vi "参数设置页.vi"() -> ()   [LabVIEW 2016, in "斯坦道总磷总氮.lvlib"]
uses:
  <vilib>/Plasmionique/MB Master/MB_Master/MB_Master.lvclass
  <vilib>/ptbypt/NI_PtbyPt.lvlib
panel:
  in  "简易流程周期设置":cluster{"switch button":bool, "设置按钮":bool}
  in  "维护模式":bool=TRUE
  out "连接状态":bool
  in  "标样核查自动补测":bool caption="通讯连接"
  in  "跨度核查自动补测":bool caption="通讯连接"
  in  "零点核查自动补测":bool caption="通讯连接"
  in  "标样核查标液偏差":dbl caption="标样核查标液偏差："
  in  "跨度核查标液偏差":dbl caption="跨度核查标液偏差："
  in  "零点核查标液偏差":dbl caption="零点核查标液偏差："
  out "低量程上限":dbl caption="低量程上限："
  in  "简易流程路径":path=path "data/流程.xml"
  out "数据刷新时间":string
  in  "通讯连接":bool=TRUE
  out "MB table":enum32{"Serial", "TCP"}(tab)
  in  "请选择串口:":refnum<visa-resource-name>
  in  "IP":string="127.0.0.1"
  in  "PORT":string="1001"
  in  "通信方式选择":enum16{"串口", "TCP"}(ring)
  in  "盐度自动补偿：":bool
  out "盐度补偿值":dbl caption="盐度补偿值："
  in  "刷新":bool
  in  "测量模式":T1(ring)
  in  "参数下拉列表":u16(ring)
  in  "量程下拉列表":enum16{"低量程", "高量程"}(ring)
  in  "测试流程路径":path=path "data/流程.xml"
  in  "标样核查量程模式":T2 caption="标样核查："
  in  "加标回收量程模式":T2 caption="加标回收："
  in  "跨度核查量程模式":T2 caption="跨度核查："
  in  "零点核查量程模式":T2 caption="零点核查："
  in  "水样测试量程模式":T2 caption="水样测试："
  out "稀释度":dbl caption="稀释度："
  out "阈值（高->低）":dbl caption="阈值（高->低）："
  out "阈值（低->高）":dbl caption="阈值（低->高）："
  out "量程下限":dbl caption="量程下限："
  out "高量程上限":dbl caption="高量程上限："
  out "检出限":dbl caption="检出限："
  out "曲线截距":dbl caption="曲线截距：" format="%#.6f"
  out "曲线斜率":dbl caption="曲线斜率：" format="%#.6f"
  out "二次多项式系数":dbl caption="二次多项式系数：" format="%#.6f"
  out "消解时长":dbl caption="消解时长："
  out "消解温度":dbl caption="消解温度："
  out "测量精度":u16 caption="测量精度："
  in  "标样核查标液浓度":dbl caption="标样核查标液浓度："
  in  "跨度核查标液浓度":dbl caption="跨度核查标液浓度："
  in  "零点核查标液浓度":dbl caption="零点核查标液浓度："
  in  "跨度值":dbl caption="跨度值："
  # "日质控设置"
  # "关键参数"
  # "连接设置"
  # "mg/L"
  # "mg/L"
  # "mg/L"
  # "mg/L"
  # "±"
  # "%"
  # "%"
  # "流程设置"
  # "简易流程周期设置"
  # "自动测试量程设置"
  # "设置："
  # "mg/L"
  # "ppt"
  # "mg/L"
  # "mg/L"
  # "mg/L"
  # "mg/L"
  # "mg/L"
  # "min"
  # "℃"
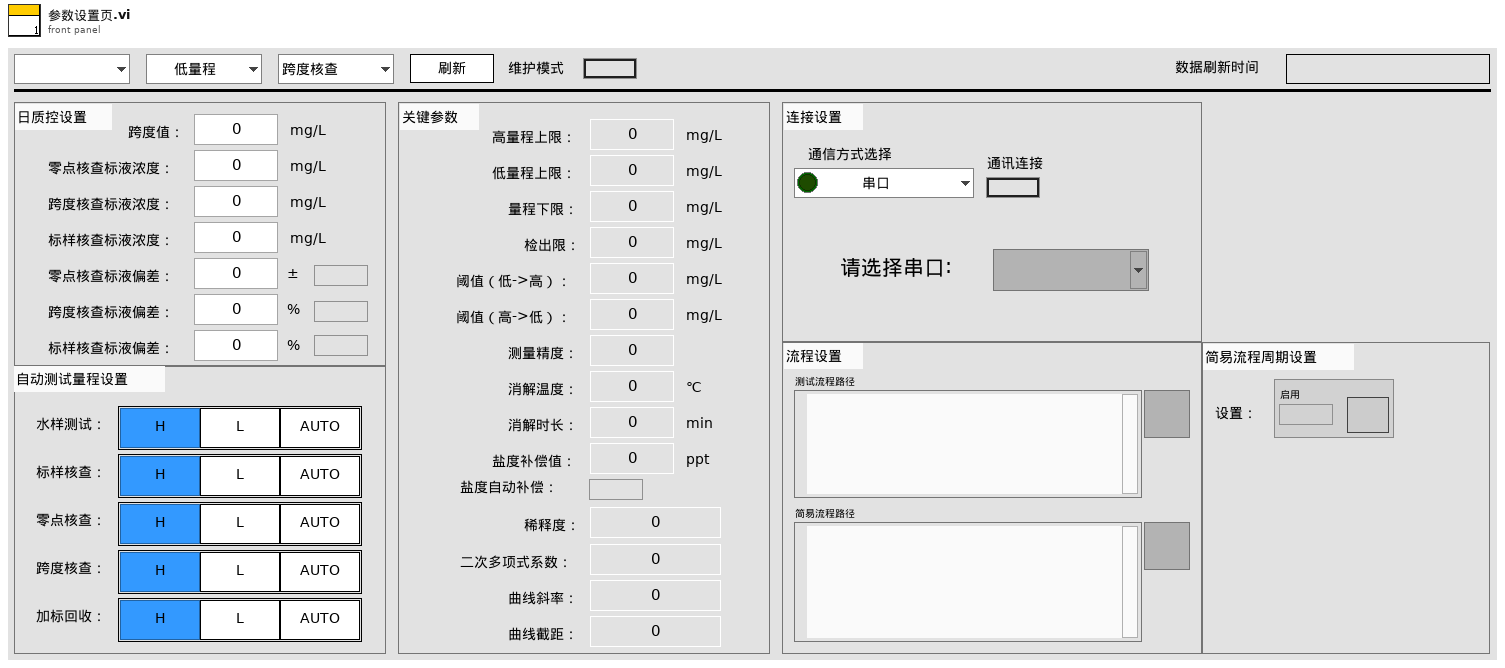
[diagram p1: front panel]
types:
  T1 = enum16{"跨度核查", "水样测量", "零点核查", "标样核查", "加标回收", "快捷测试", "空白校准", "标样校准"}
  T2 = typedef "斯坦道总磷总氮.lvlib/量程模式.ctl" = enum32{"H", "L", "AUTO"}
  T3 = typedef "Cleaning cycle.lvclass/周期项.ctl" = cluster{"时":i32, "分":i32, "频次":string, "id":i32, "参数":string, "simpleflowid":i32, "简易流程名称":string}
  T4 = cluster{"系统时间":timestamp, "工作状态":u16, "测量模式":enum16{"待机", "连续模式", "周期模式", "定点模式", "受控模式", "手动模式"}, "告警代码":u16, "故障代码":u16, "日志代码":u16, "软件版本":u16, "F0":sgl, "F1":sgl, "F2":sgl, "F3":sgl, "T":sgl, "H":sgl, "id":u16, "flowid":u16, "量程":u16, "总磷控温温度1":sgl, "营养盐控温温度2":sgl, "ADC":sgl}
  T5 = typedef "LVStringsAndValuesArrayTypeDef_U16.ctl" = cluster{"String":string, "Value":u16}[]
  T6 = enum8{"Enabled", "Disabled", "Disabled and Grayed Out"}
  T7 = cluster{"测量精度":u16, "检出限":dbl, "上限":dbl, "下限":dbl, "阈值（低->高）":dbl, "阈值（高->低）":dbl, "稀释度":dbl}
  T8 = typedef "操作日志字段定义.ctl" = cluster{"时间":timestamp, "参数":string, "日志信息":string, "流程参数":string}
  T9 = typedef "斯坦道总磷总氮.lvlib/V3 A版外设参数.ctl" = cluster{"泵类型":u8, "进样速度":u32, "出样速度":u32, "泵阀量":u8, "阀方向":u8, "光谱仪类型":u8, "光谱采样次数":u8, "氙灯次数":u8, "B":u16, "C":u16, "D":u16, "E":u16, "B_COD":u16, "C_COD":u16, "D_COD":u16, "E_COD":u16, "G":u16, "M":u16, "N":u16, "氨氮注射泵控温下限":sgl, "氨氮注射泵控温上限":sgl, "总氮注射泵控温下限":sgl, "总氮注射泵控温上限":sgl, "消解温度下限":sgl, "消解温度上限":sgl, "加热10s限值":sgl, "KP":sgl, "KI":sgl, "KD":sgl, "高温高压阀开阀温度":sgl, "总氮x公式0":u8, "总氮x公式1":sgl, "总氮x公式2":sgl, "总磷浊度稀释系数":sgl, "总磷浊度补偿权重1":sgl, "总磷浊度补偿权重2":sgl, "盐度系数":sgl, "氨氮补偿系数1":sgl, "氨氮补偿系数2":sgl}
  T10 = cluster{"水样测试量程模式":T2, "零点核查量程模式":T2, "跨度核查量程模式":T2, "加标回收量程模式":T2, "标样核查量程模式":T2}
  T11 = cluster{"总磷":dbl, "总氮":dbl, "氨氮":dbl, "磷酸盐":dbl, "硝氮":dbl, "亚硝氮":dbl, "硅酸盐":dbl, "硫化物":dbl, "COD":dbl, "氟化物":dbl, "CODMn":dbl}
  T12 = cluster{"总磷跨度值":dbl, "总磷零点标准液浓度":dbl, "总磷跨度标准液浓度":dbl, "总磷标准液标准浓度":dbl, "总氮跨度值":dbl, "总氮零点标准液浓度":dbl, "总氮跨度标准液浓度":dbl, "总氮标准液标准浓度":dbl, "COD跨度值":dbl, "COD零点标准液浓度":dbl, "COD跨度标准液浓度":dbl, "COD标准液标准浓度":dbl, "氨氮跨度值":dbl, "氨氮零点标准液浓度":dbl, "氨氮跨度标准液浓度":dbl, "氨氮标准液标准浓度":dbl, "磷酸盐跨度值":dbl, "磷酸盐零点标准液浓度":dbl, "磷酸盐跨度标准液浓度":dbl, "磷酸盐标准液标准浓度":dbl, "硝氮跨度值":dbl, "硝氮零点标准液浓度":dbl, "硝氮跨度标准液浓度":dbl, "硝氮标准液标准浓度":dbl, "亚硝氮跨度值":dbl, "亚硝氮零点标准液浓度":dbl, "亚硝氮跨度标准液浓度":dbl, "亚硝氮标准液标准浓度":dbl, "硫化物跨度值":dbl, "硫化物零点标准液浓度":dbl, "硫化物跨度标准液浓度":dbl, "硫化物标准液标准浓度":dbl, "硅酸盐跨度值":dbl, "硅酸盐零点标准液浓度":dbl, "硅酸盐跨度标准液浓度":dbl, "硅酸盐标准液标准浓度":dbl, "总磷零点标准液偏差":dbl, "总磷跨度标准液偏差":dbl, "总磷标准液标准偏差":dbl, "总氮零点标准液偏差":dbl, "总氮跨度标准液偏差":dbl, "总氮标准液标准偏差":dbl, "COD零点标准液偏差":dbl, "COD跨度标准液偏差":dbl, "COD标准液标准偏差":dbl, "氨氮零点标准液偏差":dbl, "氨氮跨度标准液偏差":dbl, "氨氮标准液标准偏差":dbl, "磷酸盐零点标准液偏差":dbl, "磷酸盐跨度标准液偏差":dbl, "磷酸盐标准液标准偏差":dbl, "硝氮零点标准液偏差":dbl, "硝氮跨度标准液偏差":dbl, "硝氮标准液标准偏差":dbl, "亚硝氮零点标准液偏差":dbl, "亚硝氮跨度标准液偏差":dbl, "亚硝氮标准液标准偏差":dbl, "硫化物零点标准液偏差":dbl, "硫化物跨度标准液偏差":dbl, "硫化物标准液标准偏差":dbl, "硅酸盐零点标准液偏差":dbl, "硅酸盐跨度标准液偏差":dbl, "硅酸盐标准液标准偏差":dbl, "氟化物跨度值":dbl, "氟化物零点标准液浓度":dbl, "氟化物跨度标准液浓度":dbl, "氟化物标准液标准浓度":dbl, "氟化物零点标准液偏差":dbl, "氟化物跨度标准液偏差":dbl, "氟化物标准液标准偏差":dbl, "CODMn跨度值":dbl, "CODMn零点标准液浓度":dbl, "CODMn跨度标准液浓度":dbl, "CODMn标准液标准浓度":dbl, "CODMn零点标准液偏差":dbl, "CODMn跨度标准液偏差":dbl, "CODMn标准液标准偏差":dbl}
  T13 = typedef "SingleStepTestV3.lvlib/SingleStepTestV3.lvclass/仪器版本.ctl" = enum16{"A版", "B版", "A1版"}
  T14 = typedef "斯坦道总磷总氮.lvlib/V3 B版外设参数.ctl" = cluster{"泵类型":u8, "注射泵正常速度":u32, "注射泵慢速":u32, "阀型号":u8, "res":u8, "光谱仪类型":u8, "光谱采样次数":u8, "氙灯次数":u8, "B":u16, "C":u16, "D":u16, "E":u16, "B_COD":u16, "C_COD":u16, "D_COD":u16, "E_COD":u16, "G":u16, "M":u16, "N":u16, "降温下限":sgl, "降温上限":sgl, "恒温温度下限":sgl, "恒温温度上限":sgl, "消解温度下限":sgl, "消解温度上限":sgl, "加热10s限值":sgl, "KP":sgl, "KI":sgl, "KD":sgl, "高温高压阀开阀温度":sgl, "总氮x公式0":u8, "总氮x公式1":sgl, "总氮x公式2":sgl, "总磷浊度稀释系数":sgl, "总磷浊度补偿权重1":sgl, "总磷浊度补偿权重2":sgl, "盐度系数":sgl, "氨氮补偿系数1":sgl, "氨氮补偿系数2":sgl, "缺试剂传感器阈值":u16}
  T15 = typedef "斯坦道总磷总氮.lvlib/V3 A1版外设参数.ctl" = cluster{"泵类型":u8, "进样速度":u32, "出样速度":u32, "泵阀量":u8, "光谱仪类型":u8, "光谱采样次数":u8, "氙灯次数":u8, "B":u16, "C":u16, "D":u16, "E":u16, "B_COD":u16, "C_COD":u16, "D_COD":u16, "E_COD":u16, "G":u16, "M":u16, "N":u16, "氨氮注射泵控温下限":sgl, "氨氮注射泵控温上限":sgl, "总氮注射泵控温下限":sgl, "总氮注射泵控温上限":sgl, "消解温度下限":sgl, "消解温度上限":sgl, "加热10s限值":sgl, "高温高压阀开阀温度":sgl, "总氮x公式0":u8, "总氮x公式1":sgl, "总氮x公式2":sgl, "总磷浊度稀释系数":sgl, "总磷浊度补偿权重1":sgl, "总磷浊度补偿权重2":sgl, "盐度系数":sgl, "氨氮补偿系数1":sgl, "氨氮补偿系数2":sgl}
  T16 = cluster{"水样测试量程模式":enum16{"H", "L", "AUTO"}, "空白核查量程模式":enum16{"H", "L", "AUTO"}, "跨度核查量程模式":enum16{"H", "L", "AUTO"}, "加标回收量程模式":enum16{"H", "L", "AUTO"}, "标样核查量程模式":enum16{"H", "L", "AUTO"}}
  T17 = cluster{"水样测试量程模式":u16, "空白核查量程模式":u16, "跨度核查量程模式":u16, "加标回收量程模式":u16, "标样核查量程模式":u16}
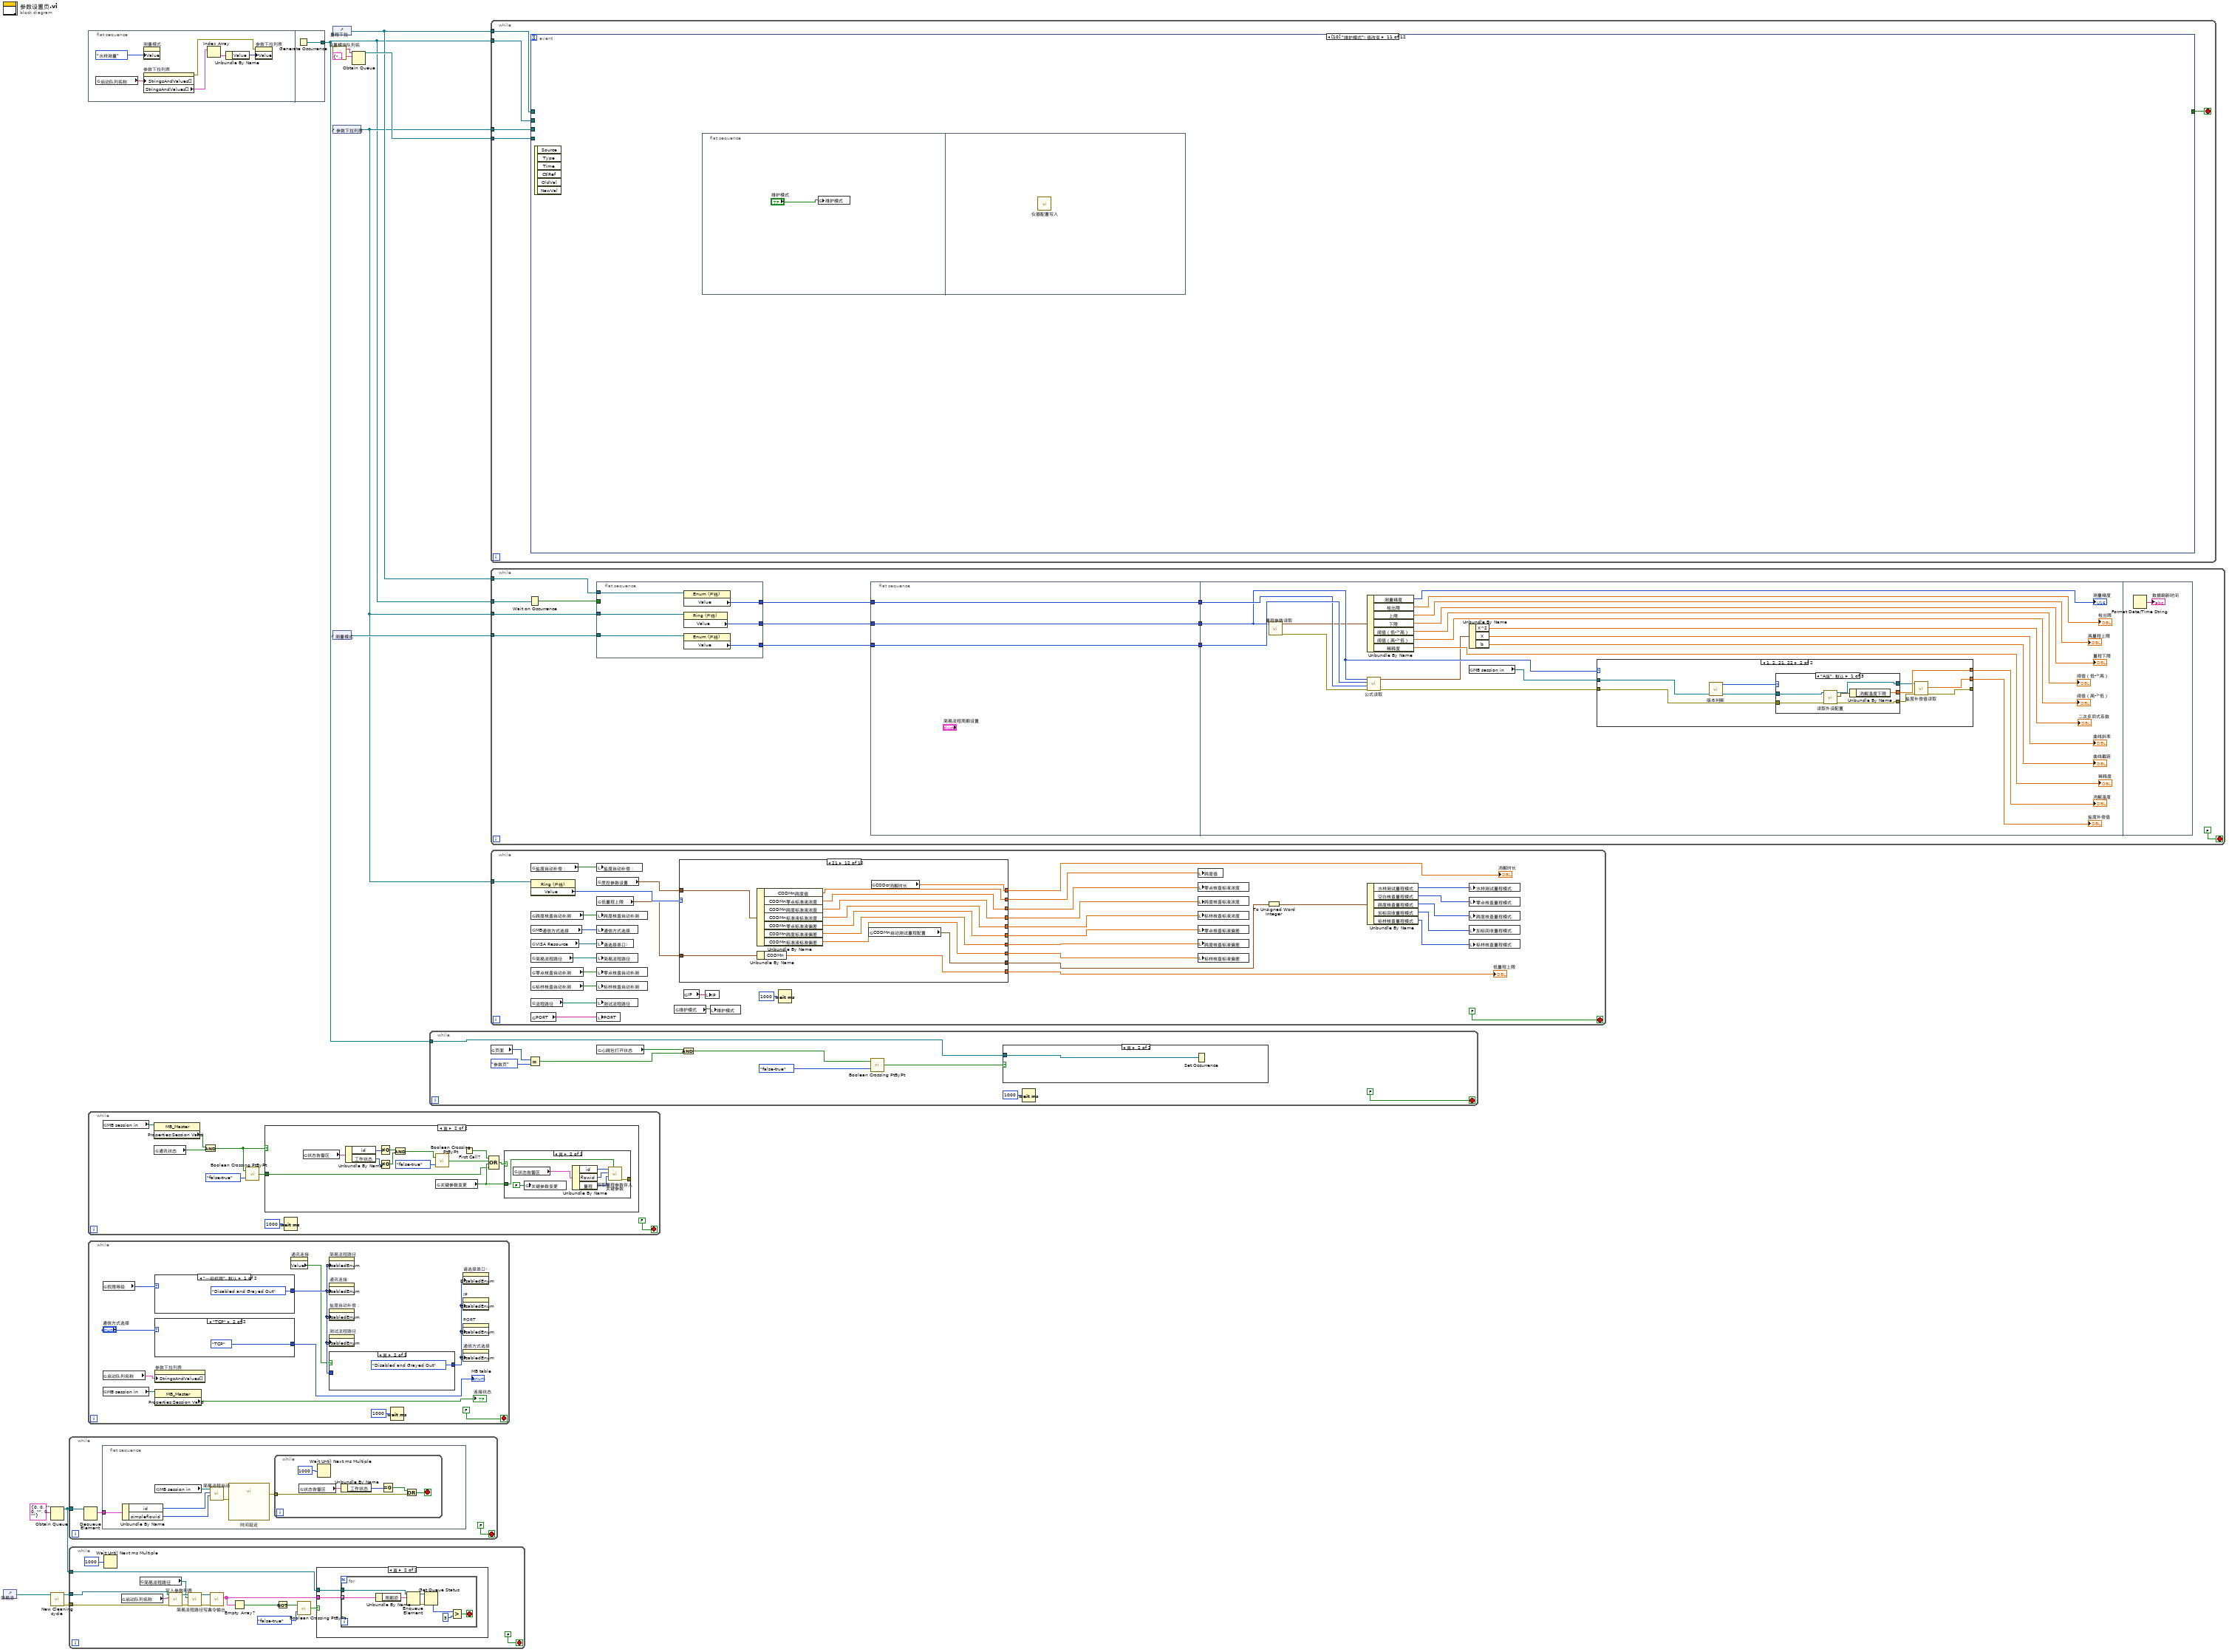
[diagram p0: block diagram]
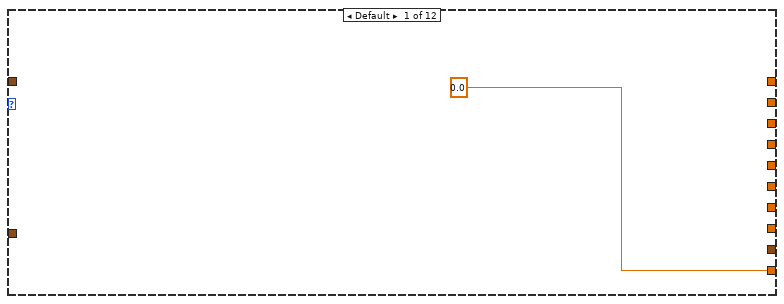
[diagram p6: hidden frame]
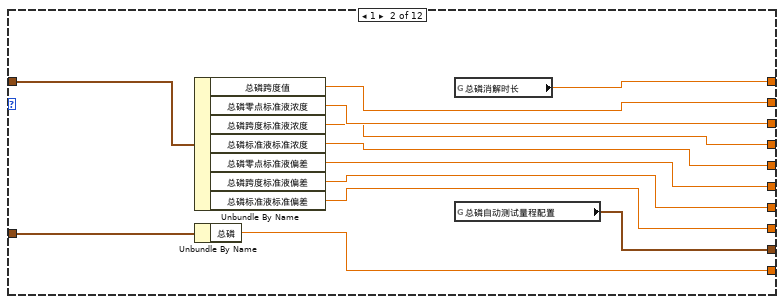
[diagram p7: hidden frame]
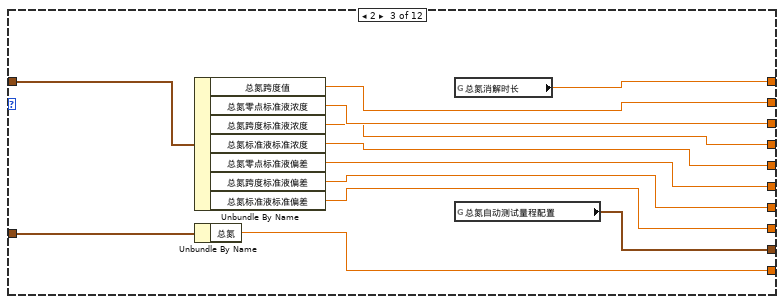
[diagram p8: hidden frame]
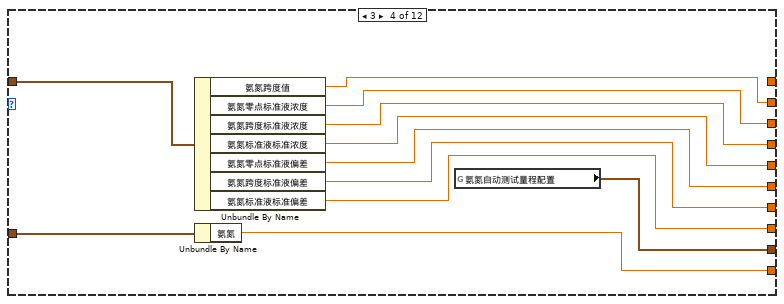
[diagram p9: hidden frame]
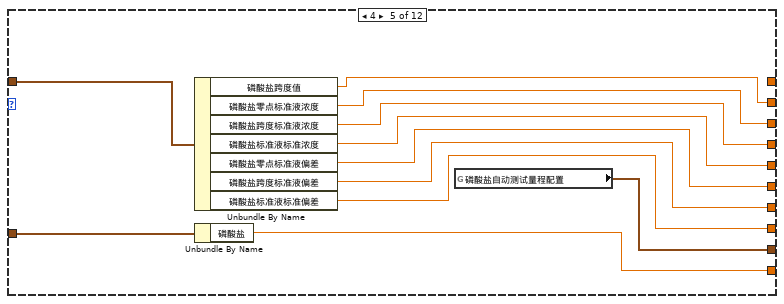
[diagram p10: hidden frame]
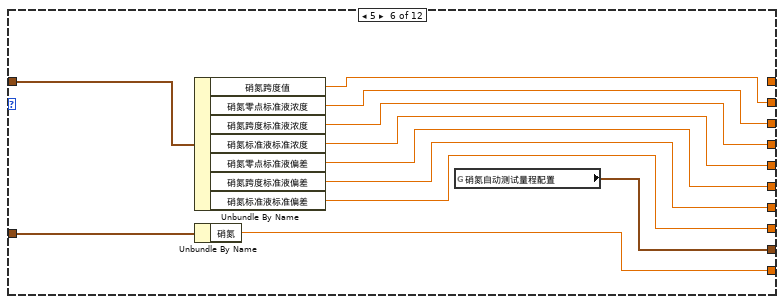
[diagram p11: hidden frame]
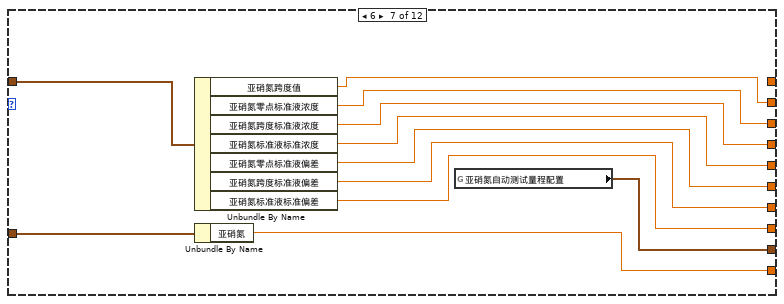
[diagram p12: hidden frame]
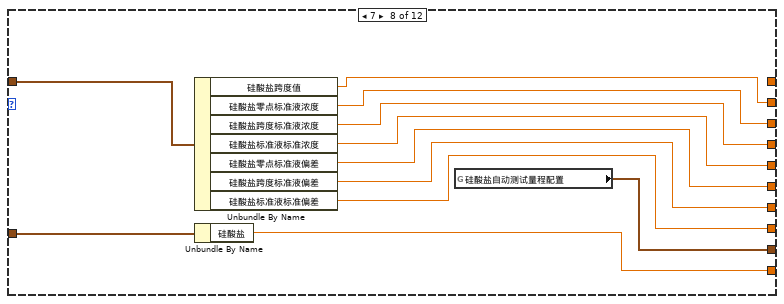
[diagram p13: hidden frame]
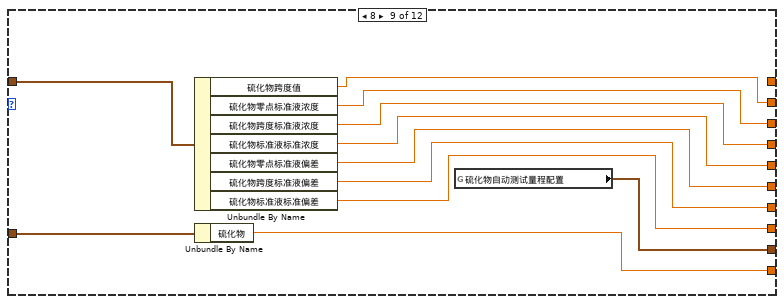
[diagram p14: hidden frame]
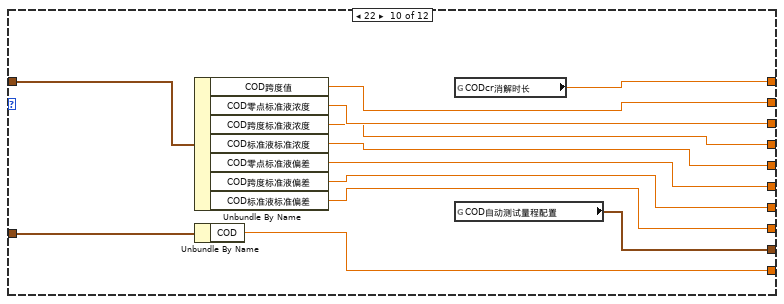
[diagram p15: hidden frame]
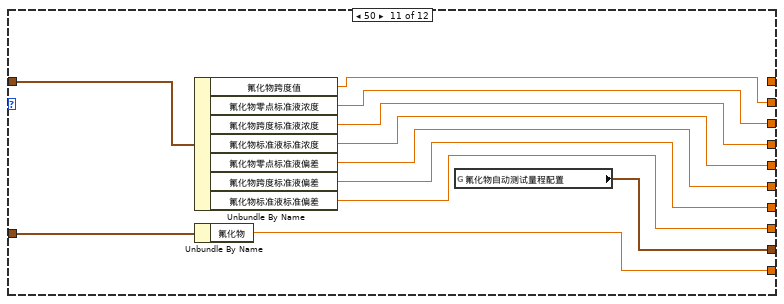
[diagram p16: hidden frame]
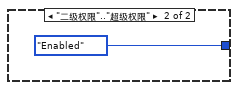
[diagram p17: hidden frame]
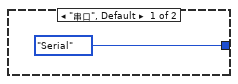
[diagram p18: hidden frame]
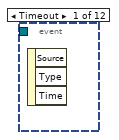
[diagram p20: hidden frame]
diagram:
  n1 = control-ref of="简易流程周期设置"() -> (w3:refnum<vi>)
  n2 = Obtain Queue(element data type=T3 {"时"=0, "分"=0, "频次"="", "id"=0, "参数"="", "simpleflowid"=0, "简易流程名称"=""} ("周期项")) -> (queue out=w1:refnum<queue>)  [unwired: 4 in, 2 out]
  n3 = call "New Cleaning cycle.vi"("Reference"=w3) -> ("error out"=w4:errorcluster, "Cleaningcycle out"=w5:refnum<class "Cleaning cycle.lvclass">)  [unwired: 9 in]
  n4 = while {
    tunnel: w1 -> [w15]
    stop <- FALSE stop-if-true
    n5 = Dequeue Element(queue=w15) -> (element=w14:T3)  [unwired: 2 in, 3 out]
    n6 = flat-sequence {
      tunnel: w14 -> [w20]
      frame #0 {
        n7 = Unbundle By Name(w20) -> ("id"=w18:i32, "simpleflowid"=w19:i32)
        n8 = global read "VAR总磷总氮全局变量.vi" "MB session in"() -> (w21:refnum<class "MB_Master.lvclass">)
        n9 = call "简易流程启动.vi"("简易流程"=w19, "参数Id"=w18, "MB session in"=w21) -> ("error out"=w17:errorcluster)  [unwired: 7 in, 1 out]
        n10 = call "时间延迟"("error in (no error)"=w17) -> ("error out"=w16:errorcluster)  [unwired: 10 in]
        n11 = while {
          tunnel: w16 -> [w23]
          stop <- w22 stop-if-true
          n12 = global read "VAR总磷总氮全局变量.vi" "状态告警区"() -> (w26:T4)
          n13 = Wait Until Next ms Multiple(millisecond multiple=u32 1000 ("毫秒倍数")) -> ()  [unwired: 1 out]
          n14 = Unbundle By Name(w26) -> ("工作状态"=w25:u16)
          n15 = Equal To 0?(x=w25) -> (x = 0?=w24:bool)
          n16 = Or(x=w24, y=w23) -> (x .or. y?=w22:bool)
        }
      }
    }
  }
  n17 = while {
    tunnel: w5 -> [w43]
    tunnel: w4 -> [w42]
    tunnel: w1 -> [w29]
    stop <- FALSE stop-if-true
    n18 = Wait Until Next ms Multiple(millisecond multiple=u32 1000 ("毫秒倍数")) -> ()  [unwired: 1 out]
    n19 = global read "model config var.vi" "启动队列名称"() -> (w39:cluster{"String":string, "Value":u16}[])
    n20 = global read "总磷总氮断电保存全局变量.vi" "简易流程路径"() -> (w38:path)
    n21 = call "写入参数列表.vi"("error in (no error)"=w42, "参数列表"=w39, "Cleaningcycle 输入"=w43) -> ("error out"=w41:errorcluster, "Cleaningcycle 输出"=w40:refnum<class "Cleaning cycle.lvclass">)  [unwired: 7 in]
    n22 = call "简易流程路径写入.vi"("error in (no error)"=w41, "简易流程路径"=w38, "Cleaningcycle 输入"=w40) -> ("error out"=w36:errorcluster, "Cleaningcycle 输出"=w37:refnum<class "Cleaning cycle.lvclass">)  [unwired: 7 in]
    n23 = call "命令输出.vi"("error in (no error)"=w36, "Cleaningcycle 输入"=w37) -> ("命令"=w31:cluster{"触发":bool, "周期项":T3}[])  [unwired: 7 in, 2 out]
    n24 = Empty Array?(array=w31) -> (empty?=w35:bool)
    n25 = Not(x=w35) -> (.not. x?=w34:bool)
    n26 = call <vilib>:"Boolean Crossing PtByPt.vi"("direction"=enum16{"either", "false-true", "true-false"}."false-true", "input"=w34) -> ("crossing"=w32:bool)  [unwired: 1 in]
    n27 = case shown="真" w32 {
      tunnel: w31 -> [_ w45]
      tunnel: w29 -> [_ w44]
      frame False {
      }
      frame True {
        n28 = for {
          tunnel: w45 -> [w53] mode=indexing
          tunnel: w44 -> [w51]
          stop <- w46 stop-if-true
          n29 = Unbundle By Name(w53) -> ("周期项"=w52:T3)
          n30 = Enqueue Element(queue=w51, element=w52) -> (queue out=w50:refnum<queue>, error out=w49:errorcluster)  [unwired: 2 in, 1 out]
          n31 = Get Queue Status(queue=w50, error in (no error)=w49) -> (# elements in queue=w48:i32)  [unwired: 1 in, 7 out]
          n32 = Greater?(x=w48, y=5) -> (0:w46:bool)
        }
      }
    }
  }
  n33 = flat-sequence {
    tunnel: [w60] -> w6
    frame #0 {
      n34 = global read "model config var.vi" "启动队列名称"() -> (w55:cluster{"String":string, "Value":u16}[])
      n35 = property on="测量模式" class="Enum (严格)"("Value"=T1."水样测量" ("测量模式")) -> ()  [unwired: 2 in, 2 out]
      n36 = property on="参数下拉列表" class="Ring (严格)"("StringsAndValues[]"=w55) -> (error out=w58:errorcluster, "StringsAndValues[]"=w56:T5)  [unwired: 2 in, 1 out]
      n37 = Index Array(array=w56) -> (element=w57:cluster{"String":string, "Value":u16})  [unwired: 1 in]
      n38 = Unbundle By Name(w57) -> ("Value"=w59:u16)
      n39 = property on="参数下拉列表" class="Ring (严格)"(error in=w58, "Value"=w59) -> ()  [unwired: 1 in, 2 out]
    }
    frame #1 {
      n40 = Generate Occurrence() -> (w60:refnum<k4>)
    }
  }
  n41 = while {
    stop <- FALSE stop-if-true
    n42 = global read "VAR总磷总氮全局变量.vi" "MB session in"() -> (w65:refnum<class "MB_Master.lvclass">)
    n43 = property class="MB_Master"(reference=w65) -> ("Properties:Session Valid"=w64:bool)  [unwired: 1 in, 2 out]
    n44 = global read "VAR总磷总氮全局变量.vi" "通讯状态"() -> (w67:bool)
    n45 = And(x=w64, y=w67) -> (x .and. y?=w62:bool)
    n46 = call <vilib>:"Boolean Crossing PtByPt.vi"("direction"=enum16{"either", "false-true", "true-false"}."false-true", "input"=w62) -> ("crossing"=w61:bool)  [unwired: 1 in]
    n47 = case shown="真" w62 {
      tunnel: w61 -> [_ w70]
      frame False {
      }
      frame True {
        n48 = global read "VAR总磷总氮全局变量.vi" "状态告警区"() -> (w80:T4)
        n49 = Unbundle By Name(w80) -> ("id"=w74:u16, "工作状态"=w79:u16)
        n50 = Not Equal To 0?(x=w74) -> (x != 0?=w75:bool)
        n51 = Not Equal To 0?(x=w79) -> (x != 0?=w76:bool)
        n52 = And(x=w75, y=w76) -> (x .and. y?=w77:bool)
        n53 = call <vilib>:"Boolean Crossing PtByPt.vi"("direction"=enum16{"either", "false-true", "true-false"}."false-true", "input"=w77) -> ("crossing"=w73:bool)  [unwired: 1 in]
        n54 = global read "VAR总磷总氮全局变量.vi" "关键参数变更"() -> (w71:bool)
        n55 = First Call?() -> (First Call?: T/F=w69:bool)
        n56 = Compound Arithmetic op=OR ("复合运算")(w69, w73, w71, w70) -> (w72:bool)
        n57 = case shown="真" w72 {
          tunnel: [_ w87] -> _
          tunnel: w71 -> [_ w82]
          frame False {
          }
          frame True {
            n58 = global read "VAR总磷总氮全局变量.vi" "状态告警区"() -> (w86:T4)
            n59 = global write "VAR总磷总氮全局变量.vi" "关键参数变更"(FALSE ("关键参数变更")) -> ()
            n60 = Unbundle By Name(w86) -> ("id"=w85:u16, "flowid"=w84:u16, "量程"=w83:u16)
            n61 = call "获取量程参数存入关键参数.vi"("关键参数变更"=w82, "量程"=w83, "flowid"=w84, "id"=w85) -> ("error out"=w87:errorcluster)  [unwired: 7 in]
          }
        }
      }
    }
    n62 = Wait (ms)(milliseconds to wait=u32 1000 ("等待时间（毫秒）")) -> ()  [unwired: 1 out]
  }
  n63 = while {
    stop <- FALSE stop-if-true
    n64 = global read "VAR总磷总氮全局变量.vi" "权限等级"() -> (w92:enum16{"一级权限", "二级权限", "三级权限", "超级权限"})
    n65 = global read "model config var.vi" "启动队列名称"() -> (w90:cluster{"String":string, "Value":u16}[])
    n66 = global read "VAR总磷总氮全局变量.vi" "MB session in"() -> (w97:refnum<class "MB_Master.lvclass">)
    n67 = case shown="\"一级权限\", 默认" w92 {
      tunnel: [T6."Disabled and Grayed Out" ("禁用") T6."Enabled" ("禁用")] -> w91
      frame "一级权限", Default {
      }
      frame "二级权限".."超级权限" {
      }
    }
    n68 = case shown="\"TCP\"" "通信方式选择" {
      tunnel: [enum32{"Serial", "TCP"}."Serial" ("MB table") enum32{"Serial", "TCP"}."TCP" ("MB table")] -> w94
      frame "串口", Default {
      }
      frame "TCP" {
      }
    }
    "MB table" <- w94
    n69 = property on="参数下拉列表" class="Ring (严格)"("StringsAndValues[]"=w90) -> ()  [unwired: 2 in, 2 out]
    n70 = property class="MB_Master"(reference=w97) -> ("Properties:Session Valid"=→"连接状态":bool)  [unwired: 1 in, 2 out]
    n71 = property on="通讯连接" class="Bool (严格)"() -> ("Value"=w88:bool)  [unwired: 2 in, 2 out]
    n72 = property on="简易流程路径" class="Path"("DisabledEnum"=w91) -> ()  [unwired: 2 in, 2 out]
    n73 = property on="通讯连接" class="Bool (严格)"("DisabledEnum"=w91) -> ()  [unwired: 2 in, 2 out]
    n74 = property on="盐度自动补偿：" class="Bool (严格)"("DisabledEnum"=w91) -> ()  [unwired: 2 in, 2 out]
    n75 = property on="测试流程路径" class="Path"("DisabledEnum"=w91) -> ()  [unwired: 2 in, 2 out]
    n76 = case shown="真" w88 {
      tunnel: [w103 T6."Disabled and Grayed Out" ("禁用")] -> w95
      tunnel: w91 -> [w103 _]
      frame False {
      }
      frame True {
      }
    }
    n77 = Wait (ms)(milliseconds to wait=u32 1000 ("等待时间（毫秒）")) -> ()  [unwired: 1 out]
    n78 = property on="请选择串口:" class="VISAName"("DisabledEnum"=w95) -> ()  [unwired: 2 in, 2 out]
    n79 = property on="IP" class="Str"("DisabledEnum"=w95) -> ()  [unwired: 2 in, 2 out]
    n80 = property on="PORT" class="Str"("DisabledEnum"=w95) -> ()  [unwired: 2 in, 2 out]
    n81 = property on="通信方式选择" class="Enum (严格)"("DisabledEnum"=w95) -> ()  [unwired: 2 in, 2 out]
  }
  n82 = control-ref of="量程下拉列表"() -> (w8:refnum<vi>)
  n83 = call "设置模块队列名.vi"() -> ("Msg"=w11:string)  [unwired: 5 in]
  n84 = control-ref of="参数下拉列表"() -> (w7:refnum<vi>)
  n85 = control-ref of="测量模式"() -> (w9:refnum<vi>)
  n86 = Obtain Queue(name (unnamed)=w11, element data type=cluster{"命令":string, "data":variant} {"命令"="", "data"=variant}) -> (queue out=w10:refnum<queue>)  [unwired: 3 in, 2 out]
  n87 = while {
    tunnel: w6 -> [w111]
    stop <- FALSE stop-if-true
    n88 = global read "VAR总磷总氮全局变量.vi" "页面"() -> (w113:enum16{"主页", "参数页", "校准页"})
    n89 = Equal?(x=w113, y=enum16{"主页", "参数页", "校准页"}."参数页" ("页面")) -> (x = y?=w112:bool)
    n90 = global read "VAR总磷总氮全局变量.vi" "心跳包打开状态"() -> (w107:bool)
    n91 = And(x=w107, y=w112) -> (x .and. y?=w108:bool)
    n92 = call <vilib>:"Boolean Crossing PtByPt.vi"("direction"=enum16{"either", "false-true", "true-false"}."false-true", "input"=w108) -> ("crossing"=w106:bool)  [unwired: 1 in]
    n93 = case shown="真" w106 {
      tunnel: w111 -> [_ w115]
      frame False {
      }
      frame True {
        n94 = Set Occurrence(w115) -> ()
      }
    }
    n95 = Wait (ms)(milliseconds to wait=u32 1000 ("等待时间（毫秒）")) -> ()  [unwired: 1 out]
  }
  n96 = while {
    tunnel: w6 -> [w119]
    tunnel: w7 -> [w118]
    tunnel: w10 -> [w117]
    tunnel: w8 -> [w116]
    stop <- w120 stop-if-true
    n97 = event shown="[10] \"维护模式\": 值改变" {
      selector: _ -> [_ _ _ _ _ _ _ _ _ _ _ _]
      dyn-events: _ -> [_ _ _ _ _ _ _ _ _ _ _ _]
      timeout: _ -> [_ _ _ _ _ _ _ _ _ _ _ _]
      tunnel: [_ TRUE _ _ _ _ _ _ _ _ _ _] -> w120
      tunnel: w119 -> [_ _ w122 _ _ _ _ _ _ w175 _ _]
      tunnel: w118 -> [_ _ _ _ w141 _ _ _ _ w177 _ _]
      tunnel: w117 -> [_ _ _ _ _ _ _ _ _ _ _ w366]
      tunnel: w116 -> [_ _ _ _ _ _ _ _ _ _ _ _]
      event Timeout {
        n98 = event-data() -> ()  [unwired: 1 in, 3 out]
      }
      event Panel Close {
        n99 = event-data() -> ()  [unwired: 1 in, 4 out]
      }
      event "参数下拉列表", "量程下拉列表", "测量模式", "刷新": Value Change {
        n100 = event-data() -> ()  [unwired: 1 in, 6 out]
        n101 = Set Occurrence(w122) -> ()
      }
      event "跨度值", "零点核查标液浓度", "跨度核查标液浓度", "标样核查标液浓度", "消解温度", "消解时长", "检出限", "高量程上限", "量程下限", "阈值（低->高）", "阈值（高->低）", "稀释度", "低量程上限", "零点核查标液偏差", "跨度核查标液偏差", "标样核查标液偏差": Mouse Down {
        n102 = event-data() -> ("CtlRef"=w124:refnum<vi>)  [unwired: 1 in, 5 out]
        n103 = global read "VAR总磷总氮全局变量.vi" "权限等级"() -> (w123:enum16{"一级权限", "二级权限", "三级权限", "超级权限"})
        n104 = case shown="\"二级权限\"..\"超级权限\"" w123 {
          tunnel: w124 -> [_ w128]
          frame "一级权限", Default {
          }
          frame "二级权限".."超级权限" {
            n105 = property class="DigNum (严格)"(reference=w128) -> (reference out=w126:refnum<vi>, "Value"=w127:dbl)  [unwired: 1 in, 1 out]
            n106 = call "数字键盘.vi"("OldNumber"=w127) -> ("NewNumber"=w125:dbl)
            n107 = property class="DigNum (严格)"(reference=w126, "Val(Sgnl)"=w125) -> ()  [unwired: 1 in, 2 out]
          }
        }
      }
      event "测量精度", "检出限", "高量程上限", "量程下限", "阈值（低->高）", "阈值（高->低）", "稀释度": Value Change {
        n108 = event-data() -> ()  [unwired: 1 in, 6 out]
        n109 = local read "测量精度"() -> (w131:u16)
        n110 = local read "检出限"() -> (w135:dbl)
        n111 = local read "高量程上限"() -> (w137:dbl)
        n112 = local read "量程下限"() -> (w136:dbl)
        n113 = local read "阈值（低->高）"() -> (w134:dbl)
        n114 = local read "阈值（高->低）"() -> (w133:dbl)
        n115 = local read "稀释度"() -> (w132:dbl)
        n116 = property class="Ring (严格)"(reference=w141) -> ("Value"=w140:u16)  [unwired: 1 in, 2 out]
        n117 = Bundle By Name(cluster=T7 {"测量精度"=0, "检出限"=0.0, "上限"=0.0, "下限"=0.0, "阈值（低->高）"=0.0, "阈值（高->低）"=0.0, "稀释度"=0.0} ("量程参数写入"), "测量精度"=w131, "检出限"=w135, "上限"=w137, "下限"=w136, "阈值（低->高）"=w134, "阈值（高->低）"=w133, "稀释度"=w132) -> (w138:T7)
        n118 = call "量程参数写入.vi"("量程参数写入"=w138, "测量参数"=w140) -> ("error out"=w129:errorcluster)  [unwired: 8 in]
        n119 = case shown="无错误" w129 {
          tunnel: ["写入成功" "写入失败"] -> w130
          frame No Error {
            n120 = Get Date/Time In Seconds() -> (seconds since 1Jan1904=w144:timestamp)
            n121 = property on="参数下拉列表" class="Ring (严格)"() -> ("RingText.Text"=w142:string)  [unwired: 2 in, 2 out]
            n122 = Bundle By Name(cluster=T8 {"时间"=timestamp(0 s since 1904-01-01), "参数"="", "日志信息"="", "流程参数"=""} ("data in"), "时间"=w144, "参数"=w142, "日志信息"="关键参数变更") -> (w145:T8)
            n123 = call "总磷总氮操作日志.vi"("data in"=w145) -> ()  [unwired: 10 in, 1 out]
            n124 = global write "VAR总磷总氮全局变量.vi" "关键参数变更"(TRUE ("关键参数变更")) -> ()
          }
          frame Error {
          }
        }
        n125 = One Button Dialog(message=w130) -> ()  [unwired: 1 in, 1 out]
      }
      event "消解温度": Value Change {
        n126 = event-data() -> ("NewVal"=w152:dbl)  [unwired: 1 in, 5 out]
        n127 = global read "VAR总磷总氮全局变量.vi" "MB session in"() -> (w153:refnum<class "MB_Master.lvclass">)
        n128 = call "读取外设配置.vi"("MB session in"=w153) -> ("error out"=w156:errorcluster, "外设配置"=w155:T9)  [unwired: 8 in, 1 out]
        n129 = Bundle By Name(cluster=w155, "消解温度下限"=w152) -> (w154:T9)
        n130 = call "写入外设配置.vi"("error in (no error)"=w156, "外设配置"=w154, "MB session in"=w153) -> ("error out"=w151:errorcluster)  [unwired: 7 in, 1 out]
        n131 = case shown="错误" w151 {
          tunnel: ["写入成功" "写入失败"] -> w150
          frame No Error {
          }
          frame Error {
          }
        }
        n132 = One Button Dialog(message=w150) -> ()  [unwired: 1 in, 1 out]
      }
      event "测量精度": Mouse Down {
        n133 = event-data() -> ("CtlRef"=w160:refnum<vi>)  [unwired: 1 in, 7 out]
        n134 = global read "VAR总磷总氮全局变量.vi" "权限等级"() -> (w159:enum16{"一级权限", "二级权限", "三级权限", "超级权限"})
        n135 = case shown="\"二级权限\"..\"超级权限\"" w159 {
          tunnel: w160 -> [_ w164]
          frame "一级权限", Default {
          }
          frame "二级权限".."超级权限" {
            n136 = property class="DigNum (严格)"(reference=w164) -> (reference out=w162:refnum<vi>, "Value"=w163:u16)  [unwired: 1 in, 1 out]
            n137 = call "数字键盘.vi"("OldNumber"=w163) -> ("NewNumber"=w161:dbl)
            n138 = property class="DigNum (严格)"(reference=w162, "Val(Sgnl)"=w161) -> ()  [unwired: 1 in, 2 out]
          }
        }
      }
      event "盐度补偿值": Mouse Down {
        n139 = event-data() -> ("CtlRef"=w166:refnum<vi>)  [unwired: 1 in, 3 out]
        n140 = global read "VAR总磷总氮全局变量.vi" "权限等级"() -> (w165:enum16{"一级权限", "二级权限", "三级权限", "超级权限"})
        n141 = case shown="\"二级权限\"..\"超级权限\"" w165 {
          tunnel: w166 -> [_ w168]
          frame "一级权限", Default {
          }
          frame "二级权限".."超级权限" {
            n142 = case shown="假" "盐度自动补偿：" {
              tunnel: w168 -> [w172 _]
              frame False {
                n143 = property class="DigNum (严格)"(reference=w172) -> (reference out=w170:refnum<vi>, "Value"=w171:dbl)  [unwired: 1 in, 1 out]
                n144 = call "数字键盘.vi"("OldNumber"=w171) -> ("NewNumber"=w169:dbl)
                n145 = property class="DigNum (严格)"(reference=w170, "Val(Sgnl)"=w169) -> ()  [unwired: 1 in, 2 out]
              }
              frame True {
              }
            }
          }
        }
      }
      event "盐度补偿值": Value Change {
        n146 = event-data() -> ("NewVal"=w173:dbl)  [unwired: 1 in, 5 out]
        n147 = global read "VAR总磷总氮全局变量.vi" "MB session in"() -> (w174:refnum<class "MB_Master.lvclass">)
        n148 = call "盐度补偿值写入.vi"("盐度补偿值"=w173, "MB session in"=w174) -> ()  [unwired: 8 in, 2 out]
      }
      event "跨度值", "零点核查标液浓度", "跨度核查标液浓度", "标样核查标液浓度", "消解时长", "测试流程路径", "盐度自动补偿：", "IP", "PORT", "请选择串口:", "通信方式选择", "简易流程路径", "低量程上限", "零点核查标液偏差", "跨度核查标液偏差", "标样核查标液偏差", "零点核查自动补测", "跨度核查自动补测", "标样核查自动补测": Value Change {
        n149 = event-data() -> ()  [unwired: 1 in, 6 out]
        n150 = global read "VAR总磷总氮全局变量.vi" "权限等级"() -> (w176:enum16{"一级权限", "二级权限", "三级权限", "超级权限"})
        n151 = case shown="\"二级权限\"..\"超级权限\"" w176 {
          tunnel: w177 -> [_ w179]
          tunnel: w175 -> [w178 _]
          frame "一级权限", Default {
            n152 = Set Occurrence(w178) -> ()
          }
          frame "二级权限".."超级权限" {
            n153 = flat-sequence {
              tunnel: w179 -> [w209]
              frame #0 {
                n154 = local read "通信方式选择"() -> (w191:enum16{"串口", "TCP"})
                n155 = property class="Ring (严格)"(reference=w209) -> ("Value"=w208:u16)  [unwired: 1 in, 2 out]
                n156 = local read "盐度自动补偿："() -> (w195:bool)
                n157 = global write "总磷总氮断电保存全局变量.vi" "MB通信方式选择"(w191) -> ()
                n158 = Bundle("水样测试量程模式"="水样测试量程模式", "零点核查量程模式"="零点核查量程模式", "跨度核查量程模式"="跨度核查量程模式", "加标回收量程模式"="加标回收量程模式", "标样核查量程模式"="标样核查量程模式") -> (w197:T10)  [unwired: 1 in]
                n159 = global write "总磷总氮断电保存全局变量.vi" "简易流程路径"("简易流程路径") -> ()
                n160 = global write "总磷总氮断电保存全局变量.vi" "IP"("IP") -> ()
                n161 = global write "总磷总氮断电保存全局变量.vi" "盐度自动补偿："(w195) -> ()
                n162 = global write "总磷总氮断电保存全局变量.vi" "流程路径"("测试流程路径") -> ()
                n163 = global write "总磷总氮断电保存全局变量.vi" "标样核查自动补测"("标样核查自动补测") -> ()
                n164 = global write "总磷总氮断电保存全局变量.vi" "PORT"("PORT") -> ()
                n165 = global write "总磷总氮断电保存全局变量.vi" "跨度核查自动补测"("跨度核查自动补测") -> ()
                n166 = global write "总磷总氮断电保存全局变量.vi" "VISA Resource"("请选择串口:") -> ()
                n167 = global write "总磷总氮断电保存全局变量.vi" "零点核查自动补测"("零点核查自动补测") -> ()
                n168 = To Unsigned Word Integer(number=w197) -> (unsigned 16bit integer=w196:cluster{u16, u16, u16, u16, u16})
                n169 = global read "总磷总氮断电保存全局变量.vi" "低量程上限"() -> (w188:T11)
                n170 = property on="低量程上限" class="DigNum (严格)"() -> ("Value"=w186:dbl)  [unwired: 2 in, 2 out]
                n171 = global read "总磷总氮断电保存全局变量.vi" "质控参数设置"() -> (w203:T12)
                n172 = local read "消解时长"() -> (w190:dbl)
                n173 = case shown="21" w208 {
                  tunnel: "跨度值" -> [_ w223 w237 w250 w263 w276 w289 w302 w315 w329 w343 w356]
                  tunnel: "标样核查标液浓度" -> [_ w220 w234 w247 w260 w273 w286 w299 w312 w326 w340 w353]
                  tunnel: "跨度核查标液浓度" -> [_ w221 w235 w248 w261 w274 w287 w300 w313 w327 w341 w354]
                  tunnel: "零点核查标液浓度" -> [_ w222 w236 w249 w262 w275 w288 w301 w314 w328 w342 w355]
                  tunnel: w203 -> [_ w225 w239 w252 w265 w278 w291 w304 w317 w331 w345 w358]
                  tunnel: w196 -> [_ w219 w233 w246 w259 w272 w285 w298 w311 w324 w338 w352]
                  tunnel: w190 -> [_ w218 w232 _ _ _ _ _ _ w325 w339 _]
                  tunnel: w188 -> [w211 w216 w231 w245 w258 w271 w284 w297 w310 w323 w337 w351]
                  tunnel: [w211 w215 w229 w244 w257 w270 w283 w296 w309 w322 w336 w350] -> w187
                  tunnel: w186 -> [_ w217 w230 w243 w256 w269 w282 w295 w308 w321 w335 w349]
                  tunnel: "标样核查标液偏差" -> [_ w214 w226 w240 w253 w268 w279 w292 w305 w318 w332 w346]
                  tunnel: "跨度核查标液偏差" -> [_ w213 w227 w241 w254 w267 w280 w293 w306 w319 w333 w347]
                  tunnel: "零点核查标液偏差" -> [_ w212 w228 w242 w255 w266 w281 w294 w307 w320 w334 w348]
                  frame 0, Default {
                  }
                  frame 1 {
                    n174 = global write "总磷总氮断电保存全局变量.vi" "总磷自动测试量程配置"(w219) -> ()
                    n175 = global write "总磷总氮断电保存全局变量.vi" "总磷消解时长"(w218) -> ()
                    n176 = Bundle By Name(cluster=w216, "总磷"=w217) -> (w215:T11)
                    n177 = Bundle By Name(cluster=w225, "总磷跨度值"=w223, "总磷零点标准液浓度"=w222, "总磷跨度标准液浓度"=w221, "总磷标准液标准浓度"=w220, "总磷零点标准液偏差"=w212, "总磷跨度标准液偏差"=w213, "总磷标准液标准偏差"=w214) -> (w224:T12)
                    n178 = global write "总磷总氮断电保存全局变量.vi" "质控参数设置"(w224) -> ()
                  }
                  frame 2 {
                    n179 = global write "总磷总氮断电保存全局变量.vi" "总氮自动测试量程配置"(w233) -> ()
                    n180 = global write "总磷总氮断电保存全局变量.vi" "总氮消解时长"(w232) -> ()
                    n181 = Bundle By Name(cluster=w231, "总氮"=w230) -> (w229:T11)
                    n182 = Bundle By Name(cluster=w239, "总氮跨度值"=w237, "总氮零点标准液浓度"=w236, "总氮跨度标准液浓度"=w235, "总氮标准液标准浓度"=w234, "总氮零点标准液偏差"=w228, "总氮跨度标准液偏差"=w227, "总氮标准液标准偏差"=w226) -> (w238:T12)
                    n183 = global write "总磷总氮断电保存全局变量.vi" "质控参数设置"(w238) -> ()
                  }
                  frame 3 {
                    n184 = global write "总磷总氮断电保存全局变量.vi" "氨氮自动测试量程配置"(w246) -> ()
                    n185 = Bundle By Name(cluster=w245, "氨氮"=w243) -> (w244:T11)
                    n186 = Bundle By Name(cluster=w252, "氨氮跨度值"=w250, "氨氮零点标准液浓度"=w249, "氨氮跨度标准液浓度"=w248, "氨氮标准液标准浓度"=w247, "氨氮零点标准液偏差"=w242, "氨氮跨度标准液偏差"=w241, "氨氮标准液标准偏差"=w240) -> (w251:T12)
                    n187 = global write "总磷总氮断电保存全局变量.vi" "质控参数设置"(w251) -> ()
                  }
                  frame 4 {
                    n188 = global write "总磷总氮断电保存全局变量.vi" "磷酸盐自动测试量程配置"(w259) -> ()
                    n189 = Bundle By Name(cluster=w258, "磷酸盐"=w256) -> (w257:T11)
                    n190 = Bundle By Name(cluster=w265, "磷酸盐跨度值"=w263, "磷酸盐零点标准液浓度"=w262, "磷酸盐跨度标准液浓度"=w261, "磷酸盐标准液标准浓度"=w260, "磷酸盐零点标准液偏差"=w255, "磷酸盐跨度标准液偏差"=w254, "磷酸盐标准液标准偏差"=w253) -> (w264:T12)
                    n191 = global write "总磷总氮断电保存全局变量.vi" "质控参数设置"(w264) -> ()
                  }
                  frame 5 {
                    n192 = global write "总磷总氮断电保存全局变量.vi" "硝氮自动测试量程配置"(w272) -> ()
                    n193 = Bundle By Name(cluster=w271, "硝氮"=w269) -> (w270:T11)
                    n194 = Bundle By Name(cluster=w278, "硝氮跨度值"=w276, "硝氮零点标准液浓度"=w275, "硝氮跨度标准液浓度"=w274, "硝氮标准液标准浓度"=w273, "硝氮零点标准液偏差"=w266, "硝氮跨度标准液偏差"=w267, "硝氮标准液标准偏差"=w268) -> (w277:T12)
                    n195 = global write "总磷总氮断电保存全局变量.vi" "质控参数设置"(w277) -> ()
                  }
                  frame 6 {
                    n196 = global write "总磷总氮断电保存全局变量.vi" "亚硝氮自动测试量程配置"(w285) -> ()
                    n197 = Bundle By Name(cluster=w284, "亚硝氮"=w282) -> (w283:T11)
                    n198 = Bundle By Name(cluster=w291, "亚硝氮跨度值"=w289, "亚硝氮零点标准液浓度"=w288, "亚硝氮跨度标准液浓度"=w287, "亚硝氮标准液标准浓度"=w286, "亚硝氮零点标准液偏差"=w281, "亚硝氮跨度标准液偏差"=w280, "亚硝氮标准液标准偏差"=w279) -> (w290:T12)
                    n199 = global write "总磷总氮断电保存全局变量.vi" "质控参数设置"(w290) -> ()
                  }
                  frame 7 {
                    n200 = global write "总磷总氮断电保存全局变量.vi" "硅酸盐自动测试量程配置"(w298) -> ()
                    n201 = Bundle By Name(cluster=w297, "硅酸盐"=w295) -> (w296:T11)
                    n202 = Bundle By Name(cluster=w304, "硅酸盐跨度值"=w302, "硅酸盐零点标准液浓度"=w301, "硅酸盐跨度标准液浓度"=w300, "硅酸盐标准液标准浓度"=w299, "硅酸盐零点标准液偏差"=w294, "硅酸盐跨度标准液偏差"=w293, "硅酸盐标准液标准偏差"=w292) -> (w303:T12)
                    n203 = global write "总磷总氮断电保存全局变量.vi" "质控参数设置"(w303) -> ()
                  }
                  frame 8 {
                    n204 = global write "总磷总氮断电保存全局变量.vi" "硫化物自动测试量程配置"(w311) -> ()
                    n205 = Bundle By Name(cluster=w310, "硫化物"=w308) -> (w309:T11)
                    n206 = Bundle By Name(cluster=w317, "硫化物跨度值"=w315, "硫化物零点标准液浓度"=w314, "硫化物跨度标准液浓度"=w313, "硫化物标准液标准浓度"=w312, "硫化物零点标准液偏差"=w307, "硫化物跨度标准液偏差"=w306, "硫化物标准液标准偏差"=w305) -> (w316:T12)
                    n207 = global write "总磷总氮断电保存全局变量.vi" "质控参数设置"(w316) -> ()
                  }
                  frame 22 {
                    n208 = global write "总磷总氮断电保存全局变量.vi" "COD自动测试量程配置"(w324) -> ()
                    n209 = global write "总磷总氮断电保存全局变量.vi" "CODcr消解时长"(w325) -> ()
                    n210 = Bundle By Name(cluster=w323, "COD"=w321) -> (w322:T11)
                    n211 = Bundle By Name(cluster=w331, "COD跨度值"=w329, "COD零点标准液浓度"=w328, "COD跨度标准液浓度"=w327, "COD标准液标准浓度"=w326, "COD零点标准液偏差"=w320, "COD跨度标准液偏差"=w319, "COD标准液标准偏差"=w318) -> (w330:T12)
                    n212 = global write "总磷总氮断电保存全局变量.vi" "质控参数设置"(w330) -> ()
                  }
                  frame 21 {
                    n213 = global write "总磷总氮断电保存全局变量.vi" "CODMn自动测试量程配置"(w338) -> ()
                    n214 = global write "总磷总氮断电保存全局变量.vi" "CODmn消解时长"(w339) -> ()
                    n215 = Bundle By Name(cluster=w337, "CODMn"=w335) -> (w336:T11)
                    n216 = Bundle By Name(cluster=w345, "CODMn跨度值"=w343, "CODMn零点标准液浓度"=w342, "CODMn跨度标准液浓度"=w341, "CODMn标准液标准浓度"=w340, "CODMn零点标准液偏差"=w334, "CODMn跨度标准液偏差"=w333, "CODMn标准液标准偏差"=w332) -> (w344:T12)
                    n217 = global write "总磷总氮断电保存全局变量.vi" "质控参数设置"(w344) -> ()
                  }
                  frame 50 {
                    n218 = global write "总磷总氮断电保存全局变量.vi" "氟化物自动测试量程配置"(w352) -> ()
                    n219 = Bundle By Name(cluster=w351, "氟化物"=w349) -> (w350:T11)
                    n220 = Bundle By Name(cluster=w358, "氟化物跨度值"=w356, "氟化物零点标准液浓度"=w355, "氟化物跨度标准液浓度"=w354, "氟化物标准液标准浓度"=w353, "氟化物零点标准液偏差"=w348, "氟化物跨度标准液偏差"=w347, "氟化物标准液标准偏差"=w346) -> (w357:T12)
                    n221 = global write "总磷总氮断电保存全局变量.vi" "质控参数设置"(w357) -> ()
                  }
                }
                n222 = global write "总磷总氮断电保存全局变量.vi" "低量程上限"(w187) -> ()
              }
              frame #1 {
                n223 = Get Date/Time In Seconds() -> (seconds since 1Jan1904=w361:timestamp)
                n224 = property on="参数下拉列表" class="Ring (严格)"() -> ("RingText.Text"=w359:string)  [unwired: 2 in, 2 out]
                n225 = Bundle By Name(cluster=T8 {"时间"=timestamp(0 s since 1904-01-01), "参数"="", "日志信息"="", "流程参数"=""} ("data in"), "时间"=w361, "参数"=w359, "日志信息"="参数变更") -> (w362:T8)
                n226 = call "总磷总氮操作日志.vi"("data in"=w362) -> ()  [unwired: 10 in, 1 out]
                n227 = call "仪器配置写入.vi"() -> ()  [unwired: 11 in, 1 out]
              }
            }
          }
        }
      }
      event "维护模式": Value Change {
        n228 = event-data() -> ()  [unwired: 1 in, 6 out]
        n229 = flat-sequence {
          frame #0 {
            n230 = global write "总磷总氮断电保存全局变量.vi" "维护模式"("维护模式") -> ()
          }
          frame #1 {
            n231 = call "仪器配置写入.vi"() -> ()  [unwired: 11 in, 1 out]
          }
        }
      }
      event "通讯连接": Value Change {
        n232 = event-data() -> ("NewVal"=w365:bool)  [unwired: 1 in, 5 out]
        n233 = Flush Queue(queue=w366) -> (queue out=w367:refnum<queue>)  [unwired: 1 in, 2 out]
        n234 = case shown="假" w365 {
          tunnel: w367 -> [w368 w370]
          frame False {
            n235 = Enqueue Element At Opposite End(queue=w368, element=cluster{"命令":string, "data":variant} {"命令"="停用模块", "data"=variant} ("元素")) -> ()  [unwired: 2 in, 3 out]
          }
          frame True {
            n236 = Enqueue Element At Opposite End(queue=w370, element=cluster{"命令":string, "data":variant} {"命令"="启用模块", "data"=variant} ("元素")) -> ()  [unwired: 2 in, 3 out]
          }
        }
      }
    }
  }
  n237 = while {
    tunnel: w7 -> [w382]
    tunnel: w8 -> [w381]
    tunnel: w9 -> [w380]
    tunnel: w6 -> [w379]
    stop <- FALSE stop-if-true
    n238 = Wait on Occurrence(2:w379) -> (0:w373:bool)  [unwired: 2 in]
    n239 = flat-sequence {
      tunnel: w382 -> [w389]
      tunnel: w381 -> [w388]
      tunnel: w380 -> [w387]
      tunnel: [w386] -> w376
      tunnel: [w385] -> w375
      tunnel: [w384] -> w374
      tunnel: w373 -> [_]
      frame #0 {
        n240 = property class="Enum (严格)"(reference=w388) -> ("Value"=w385:enum16{"低量程", "高量程"})  [unwired: 1 in, 2 out]
        n241 = property class="Ring (严格)"(reference=w389) -> ("Value"=w386:u16)  [unwired: 1 in, 2 out]
        n242 = property class="Enum (严格)"(reference=w387) -> ("Value"=w384:T1)  [unwired: 1 in, 2 out]
      }
    }
    n243 = flat-sequence {
      tunnel: [w392] -> w378
      tunnel: [w391] -> w377
      tunnel: w376 -> [w390]
      tunnel: w375 -> [w392]
      tunnel: w374 -> [w391]
      tunnel: [w390] -> w372
      tunnel: w378 -> [w411]
      tunnel: w377 -> [w412]
      tunnel: w372 -> [w410]
      frame #0 {
      }
      frame #1 {
        n244 = call "量程参数读取.vi"("测量参数"=w410) -> ("error out"=w401:errorcluster, "量程参数读取"=w409:T7)  [unwired: 9 in]
        n245 = Unbundle By Name(w409) -> ("测量精度"=→"测量精度":u16, "检出限"=→"检出限":dbl, "上限"=→"高量程上限":dbl, "下限"=→"量程下限":dbl, "阈值（低->高）"=→"阈值（低->高）":dbl, "阈值（高->低）"=→"阈值（高->低）":dbl, "稀释度"=→"稀释度":dbl)
        n246 = call "公式读取.vi"("error in (no error)"=w401, "量程"=w411, "测量模式"=w412, "测量参数"=w410) -> ("error out"=w395:errorcluster, "公式"=w400:cluster{"X^2":dbl, "X":dbl, "b":dbl})  [unwired: 6 in]
        n247 = Unbundle By Name(w400) -> ("X^2"=→"二次多项式系数":dbl, "X"=→"曲线斜率":dbl, "b"=→"曲线截距":dbl)
        n248 = global read "VAR总磷总氮全局变量.vi" "MB session in"() -> (w394:refnum<class "MB_Master.lvclass">)
        n249 = case shown="1, 2, 21, 22" w410 {
          tunnel: [_ w415] -> w396
          tunnel: [w413 w421] -> _
          tunnel: w395 -> [w413 w416]
          tunnel: w394 -> [_ w419]
          tunnel: [_ w420] -> w393
          frame 0, Default {
          }
          frame 1, 2, 21, 22 {
            n250 = call "版本判断.vi"() -> ("仪器版本"=w418:T13)  [unwired: 11 in]
            n251 = case shown="\"A版\", 默认" w418 {
              tunnel: [w427 w431 w437] -> w417
              tunnel: w419 -> [w426 w432 w438]
              tunnel: [w423 w429 w435] -> w415
              tunnel: w416 -> [w425 _ w434]
              tunnel: [w422 w428 w433] -> w414
              frame "A版", Default {
                n252 = call "读取外设配置.vi"("error in (no error)"=w425, "MB session in"=w426) -> ("error out"=w427:errorcluster, "外设配置"=w424:T9, "MB session out"=w422:refnum<class "MB_Master.lvclass">)  [unwired: 7 in]
                n253 = Unbundle By Name(w424) -> ("消解温度下限"=w423:sgl)
              }
              frame "B版" {
                n254 = call "读取B版外设配置.vi"("MB session in"=w432) -> ("error out"=w431:errorcluster, "外设配置"=w430:T14, "MB session out"=w428:refnum<class "MB_Master.lvclass">)  [unwired: 8 in]
                n255 = Unbundle By Name(w430) -> ("消解温度下限"=w429:sgl)
              }
              frame "A1版" {
                n256 = call "读取A1外设配置.vi"("error in (no error)"=w434, "MB session in"=w438) -> ("error out"=w437:errorcluster, "外设配置"=w436:T15, "MB session out"=w433:refnum<class "MB_Master.lvclass">)  [unwired: 7 in]
                n257 = Unbundle By Name(w436) -> ("消解温度下限"=w435:sgl)
              }
            }
            n258 = call "盐度补偿值读取.vi"("Error in"=w417, "MB session in"=w414) -> ("error out"=w421:errorcluster, "盐度补偿值"=w420:sgl)  [unwired: 7 in, 1 out]
          }
        }
        "消解温度" <- w396
        "盐度补偿值" <- w393
      }
      frame #2 {
        n259 = Format Date/Time String() -> (date/time string=→"数据刷新时间":string)  [unwired: 3 in]
      }
    }
  }
  n260 = while {
    tunnel: w7 -> [w451]
    stop <- FALSE stop-if-true
    n261 = global read "总磷总氮断电保存全局变量.vi" "盐度自动补偿："() -> (w466:bool)
    n262 = property class="Ring (严格)"(reference=w451) -> ("Value"=w450:u16)  [unwired: 1 in, 2 out]
    n263 = global read "总磷总氮断电保存全局变量.vi" "跨度核查自动补测"() -> (w441:bool)
    n264 = global read "总磷总氮断电保存全局变量.vi" "MB通信方式选择"() -> (w465:enum16{"串口", "TCP"})
    n265 = global read "总磷总氮断电保存全局变量.vi" "VISA Resource"() -> (w470:refnum<visa-resource-name>)
    n266 = global read "总磷总氮断电保存全局变量.vi" "简易流程路径"() -> (w449:path)
    n267 = global read "总磷总氮断电保存全局变量.vi" "零点核查自动补测"() -> (w443:bool)
    n268 = global read "总磷总氮断电保存全局变量.vi" "标样核查自动补测"() -> (w442:bool)
    n269 = global read "总磷总氮断电保存全局变量.vi" "流程路径"() -> (w467:path)
    n270 = global read "总磷总氮断电保存全局变量.vi" "PORT"() -> (w469:string)
    n271 = local write "盐度自动补偿："(w466) -> ()
    n272 = global read "总磷总氮断电保存全局变量.vi" "质控参数设置"() -> (w460:T12)
    n273 = global read "总磷总氮断电保存全局变量.vi" "低量程上限"() -> (w448:T11)
    n274 = local write "跨度核查自动补测"(w441) -> ()
    n275 = local write "通信方式选择"(w465) -> ()
    n276 = local write "请选择串口:"(w470) -> ()
    n277 = local write "简易流程路径"(w449) -> ()
    n278 = local write "零点核查自动补测"(w443) -> ()
    n279 = local write "标样核查自动补测"(w442) -> ()
    n280 = local write "测试流程路径"(w467) -> ()
    n281 = local write "PORT"(w469) -> ()
    n282 = global read "总磷总氮断电保存全局变量.vi" "维护模式"() -> (w440:bool)
    n283 = case shown="21" w450 {
      tunnel: [_ w485 w497 w508 w519 w530 w541 w552 w563 w575 w586 w598] -> w458
      tunnel: [_ w484 w496 _ _ _ _ _ _ w574 _ w587] -> w459
      tunnel: w460 -> [_ w483 w495 w507 w518 w529 w540 w551 w562 w573 w585 w597]
      tunnel: [_ w482 w494 w506 w517 w528 w539 w550 w561 w572 w584 w596] -> w461
      tunnel: [_ w481 w493 w505 w516 w527 w538 w549 w560 w571 w583 w595] -> w462
      tunnel: [_ w480 w492 w504 w515 w526 w537 w548 w559 w570 w582 w594] -> w463
      tunnel: [_ w479 w491 w503 w514 w525 w536 w547 w558 w569 w581 w593] -> w464
      tunnel: w448 -> [_ w478 w490 w502 w513 w524 w535 w546 w557 w568 w580 w592]
      tunnel: [0.0 ("COD") w477 w489 w501 w512 w523 w534 w545 w556 w567 w579 w591] -> w447
      tunnel: [_ w476 w488 w500 w511 w522 w533 w544 w555 w566 w578 w590] -> w446
      tunnel: [_ w475 w487 w499 w510 w521 w532 w543 w554 w565 w577 w589] -> w445
      tunnel: [_ w474 w486 w498 w509 w520 w531 w542 w553 w564 w576 w588] -> w444
      frame Default {
      }
      frame 1 {
        n284 = Unbundle By Name(w483) -> ("总磷跨度值"=w482:dbl, "总磷零点标准液浓度"=w481:dbl, "总磷跨度标准液浓度"=w480:dbl, "总磷标准液标准浓度"=w479:dbl, "总磷零点标准液偏差"=w476:dbl, "总磷跨度标准液偏差"=w475:dbl, "总磷标准液标准偏差"=w474:dbl)
        n285 = Unbundle By Name(w478) -> ("总磷"=w477:dbl)
        n286 = global read "总磷总氮断电保存全局变量.vi" "总磷消解时长"() -> (w484:dbl)
        n287 = global read "总磷总氮断电保存全局变量.vi" "总磷自动测试量程配置"() -> (w485:T16)
      }
      frame 2 {
        n288 = Unbundle By Name(w495) -> ("总氮跨度值"=w494:dbl, "总氮零点标准液浓度"=w493:dbl, "总氮跨度标准液浓度"=w492:dbl, "总氮标准液标准浓度"=w491:dbl, "总氮零点标准液偏差"=w488:dbl, "总氮跨度标准液偏差"=w487:dbl, "总氮标准液标准偏差"=w486:dbl)
        n289 = Unbundle By Name(w490) -> ("总氮"=w489:dbl)
        n290 = global read "总磷总氮断电保存全局变量.vi" "总氮消解时长"() -> (w496:dbl)
        n291 = global read "总磷总氮断电保存全局变量.vi" "总氮自动测试量程配置"() -> (w497:T16)
      }
      frame 3 {
        n292 = Unbundle By Name(w507) -> ("氨氮跨度值"=w506:dbl, "氨氮零点标准液浓度"=w505:dbl, "氨氮跨度标准液浓度"=w504:dbl, "氨氮标准液标准浓度"=w503:dbl, "氨氮零点标准液偏差"=w500:dbl, "氨氮跨度标准液偏差"=w499:dbl, "氨氮标准液标准偏差"=w498:dbl)
        n293 = Unbundle By Name(w502) -> ("氨氮"=w501:dbl)
        n294 = global read "总磷总氮断电保存全局变量.vi" "氨氮自动测试量程配置"() -> (w508:T16)
      }
      frame 4 {
        n295 = Unbundle By Name(w518) -> ("磷酸盐跨度值"=w517:dbl, "磷酸盐零点标准液浓度"=w516:dbl, "磷酸盐跨度标准液浓度"=w515:dbl, "磷酸盐标准液标准浓度"=w514:dbl, "磷酸盐零点标准液偏差"=w511:dbl, "磷酸盐跨度标准液偏差"=w510:dbl, "磷酸盐标准液标准偏差"=w509:dbl)
        n296 = Unbundle By Name(w513) -> ("磷酸盐"=w512:dbl)
        n297 = global read "总磷总氮断电保存全局变量.vi" "磷酸盐自动测试量程配置"() -> (w519:T16)
      }
      frame 5 {
        n298 = Unbundle By Name(w529) -> ("硝氮跨度值"=w528:dbl, "硝氮零点标准液浓度"=w527:dbl, "硝氮跨度标准液浓度"=w526:dbl, "硝氮标准液标准浓度"=w525:dbl, "硝氮零点标准液偏差"=w522:dbl, "硝氮跨度标准液偏差"=w521:dbl, "硝氮标准液标准偏差"=w520:dbl)
        n299 = Unbundle By Name(w524) -> ("硝氮"=w523:dbl)
        n300 = global read "总磷总氮断电保存全局变量.vi" "硝氮自动测试量程配置"() -> (w530:T16)
      }
      frame 6 {
        n301 = Unbundle By Name(w540) -> ("亚硝氮跨度值"=w539:dbl, "亚硝氮零点标准液浓度"=w538:dbl, "亚硝氮跨度标准液浓度"=w537:dbl, "亚硝氮标准液标准浓度"=w536:dbl, "亚硝氮零点标准液偏差"=w533:dbl, "亚硝氮跨度标准液偏差"=w532:dbl, "亚硝氮标准液标准偏差"=w531:dbl)
        n302 = Unbundle By Name(w535) -> ("亚硝氮"=w534:dbl)
        n303 = global read "总磷总氮断电保存全局变量.vi" "亚硝氮自动测试量程配置"() -> (w541:T16)
      }
      frame 7 {
        n304 = Unbundle By Name(w551) -> ("硅酸盐跨度值"=w550:dbl, "硅酸盐零点标准液浓度"=w549:dbl, "硅酸盐跨度标准液浓度"=w548:dbl, "硅酸盐标准液标准浓度"=w547:dbl, "硅酸盐零点标准液偏差"=w544:dbl, "硅酸盐跨度标准液偏差"=w543:dbl, "硅酸盐标准液标准偏差"=w542:dbl)
        n305 = Unbundle By Name(w546) -> ("硅酸盐"=w545:dbl)
        n306 = global read "总磷总氮断电保存全局变量.vi" "硅酸盐自动测试量程配置"() -> (w552:T16)
      }
      frame 8 {
        n307 = Unbundle By Name(w562) -> ("硫化物跨度值"=w561:dbl, "硫化物零点标准液浓度"=w560:dbl, "硫化物跨度标准液浓度"=w559:dbl, "硫化物标准液标准浓度"=w558:dbl, "硫化物零点标准液偏差"=w555:dbl, "硫化物跨度标准液偏差"=w554:dbl, "硫化物标准液标准偏差"=w553:dbl)
        n308 = Unbundle By Name(w557) -> ("硫化物"=w556:dbl)
        n309 = global read "总磷总氮断电保存全局变量.vi" "硫化物自动测试量程配置"() -> (w563:T16)
      }
      frame 22 {
        n310 = Unbundle By Name(w573) -> ("COD跨度值"=w572:dbl, "COD零点标准液浓度"=w571:dbl, "COD跨度标准液浓度"=w570:dbl, "COD标准液标准浓度"=w569:dbl, "COD零点标准液偏差"=w566:dbl, "COD跨度标准液偏差"=w565:dbl, "COD标准液标准偏差"=w564:dbl)
        n311 = Unbundle By Name(w568) -> ("COD"=w567:dbl)
        n312 = global read "总磷总氮断电保存全局变量.vi" "CODcr消解时长"() -> (w574:dbl)
        n313 = global read "总磷总氮断电保存全局变量.vi" "COD自动测试量程配置"() -> (w575:T16)
      }
      frame 50 {
        n314 = Unbundle By Name(w585) -> ("氟化物跨度值"=w584:dbl, "氟化物零点标准液浓度"=w583:dbl, "氟化物跨度标准液浓度"=w582:dbl, "氟化物标准液标准浓度"=w581:dbl, "氟化物零点标准液偏差"=w578:dbl, "氟化物跨度标准液偏差"=w577:dbl, "氟化物标准液标准偏差"=w576:dbl)
        n315 = Unbundle By Name(w580) -> ("氟化物"=w579:dbl)
        n316 = global read "总磷总氮断电保存全局变量.vi" "氟化物自动测试量程配置"() -> (w586:T16)
      }
      frame 21 {
        n317 = Unbundle By Name(w597) -> ("CODMn跨度值"=w596:dbl, "CODMn零点标准液浓度"=w595:dbl, "CODMn跨度标准液浓度"=w594:dbl, "CODMn标准液标准浓度"=w593:dbl, "CODMn零点标准液偏差"=w590:dbl, "CODMn跨度标准液偏差"=w589:dbl, "CODMn标准液标准偏差"=w588:dbl)
        n318 = Unbundle By Name(w592) -> ("CODMn"=w591:dbl)
        n319 = global read "总磷总氮断电保存全局变量.vi" "CODMn自动测试量程配置"() -> (w598:T16)
        n320 = global read "总磷总氮断电保存全局变量.vi" "CODcr消解时长"() -> (w587:dbl)
      }
    }
    "消解时长" <- w459
    "低量程上限" <- w447
    n321 = global read "总磷总氮断电保存全局变量.vi" "IP"() -> (w468:string)
    n322 = local write "IP"(w468) -> ()
    n323 = local write "维护模式"(w440) -> ()
    n324 = Wait (ms)(milliseconds to wait=u32 1000 ("等待时间（毫秒）")) -> ()  [unwired: 1 out]
    n325 = local write "跨度值"(w461) -> ()
    n326 = local write "零点核查标液浓度"(w462) -> ()
    n327 = local write "跨度核查标液浓度"(w463) -> ()
    n328 = local write "标样核查标液浓度"(w464) -> ()
    n329 = local write "零点核查标液偏差"(w446) -> ()
    n330 = local write "跨度核查标液偏差"(w445) -> ()
    n331 = local write "标样核查标液偏差"(w444) -> ()
    n332 = To Unsigned Word Integer(number=w458) -> (unsigned 16bit integer=w457:T17)
    n333 = Unbundle By Name(w457) -> ("水样测试量程模式"=w456:u16, "空白核查量程模式"=w454:u16, "跨度核查量程模式"=w453:u16, "加标回收量程模式"=w452:u16, "标样核查量程模式"=w455:u16)
    n334 = local write "水样测试量程模式"(w456) -> ()
    n335 = local write "零点核查量程模式"(w454) -> ()
    n336 = local write "跨度核查量程模式"(w453) -> ()
    n337 = local write "加标回收量程模式"(w452) -> ()
    n338 = local write "标样核查量程模式"(w455) -> ()
  }
